vi "read_udc_continuous.vi"(1 "Hex Address":u16 format="%x", 2 "TCP Connection Refnum in":refnum<k5>) -> (0 "Value":dbl)   [LabVIEW 2011]
uses:
  <vilib>/NI Modbus.llb/MB Ethernet Master Query Read Input Registers (poly).vi
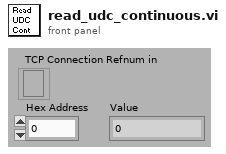
[diagram p1: front panel]
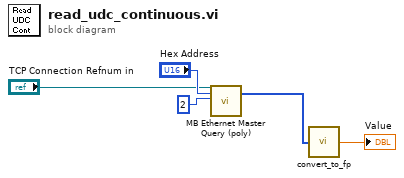
[diagram p0: block diagram]
diagram:
  n1 = call-poly <vilib>:"MB Ethernet Master Query (poly).vi"("TCP Connection Refnum in"="TCP Connection Refnum in", "Starting Address"="Hex Address", "Quantity"=u16 2) -> ("Input Registers"=w4:u16[])  [unwired: 2 in, 14 out]
  n2 = call "convert_to_fp.vi"("Input Array"=w4) -> ("Floating point"=→"Value":sgl)
